vi "Main.vi"() -> ()   [LabVIEW 8.6]
uses:
  <vilib>/Analysis/NI_AALBase.lvlib
  <vilib>/Analysis/baseanly.llb/Mean (DBL).vi
panel:
  out "TemplateFilePath":path
  in  "Inspectors":string
  out "AvgValue":dbl
  out "CurveGraph":dbl[](graph)
  in  "Standard":string
  in  "SN":string
  in  "Type":string
  out "DateTime":timestamp format="%<%H:%M\n%Y/%m/%d>T"
  # "請看程式區說明"
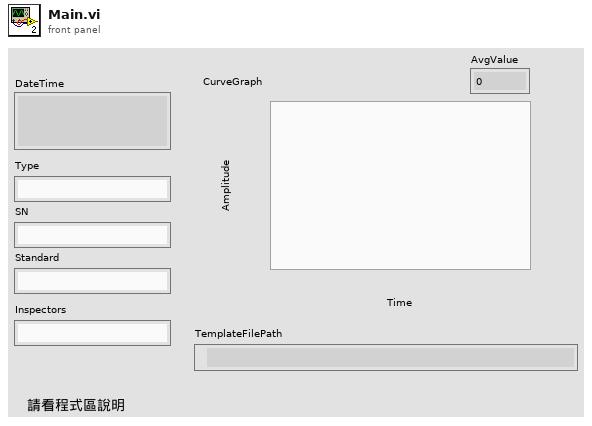
[diagram p1: front panel]
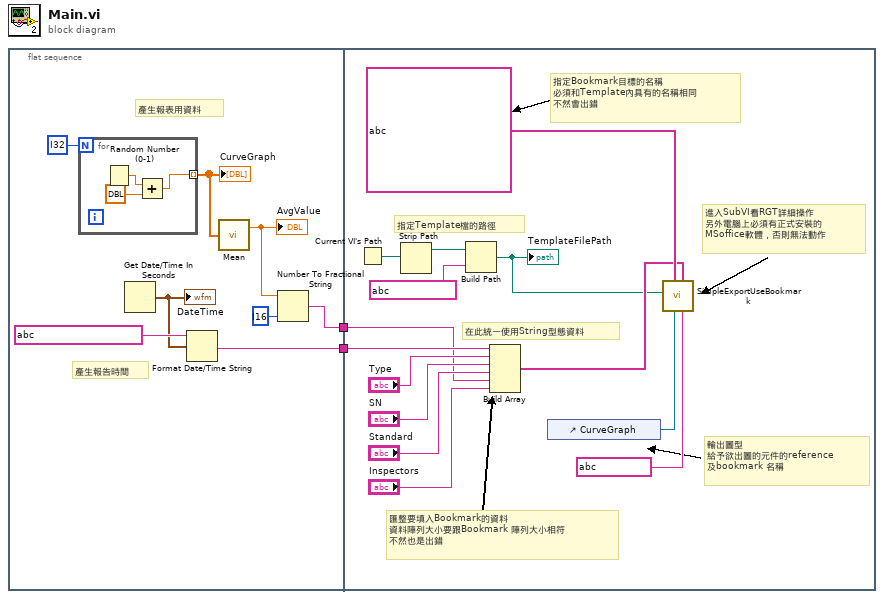
[diagram p0: block diagram]
diagram:
  n1 = flat-sequence {
    tunnel: [w4] -> w2
    tunnel: [w3] -> w1
    tunnel: w2 -> [w26]
    tunnel: w1 -> [w22]
    frame #0 {
      # "產生報告時間"
      # "產生報表用資料"
      n2 = for {
        N: i32 ? ("Numeric") -> [_]
        tunnel: [w11] -> w9 mode=indexing
        n3 = Random Number (0-1)() -> (number: 0 to 1=w13:dbl)
        n4 = Add(x=w13, y=dbl ?) -> (x+y=w11:dbl)
      }
      "CurveGraph" <- w9
      n5 = Get Date/Time In Seconds() -> (seconds since 1Jan1904=w7:timestamp)
      "DateTime" <- w7
      n6 = Format Date/Time String(time format string (%c)=string ?, seconds (now)=w7) -> (date/time string=w4:string)  [unwired: 1 in]
      n7 = call-poly <vilib>:"Mean.vi"("X"=w9) -> ("mean"=w6:dbl)  [unwired: 1 out]
      "AvgValue" <- w6
      n8 = Number To Fractional String(number=w6, precision (6)=i16 ?) -> (F-format string=w3:string)  [unwired: 2 in]
    }
    frame #1 {
      # "在此統一使用String型態資料"
      # "進入SubVI看RGT詳細操作\n另外電腦上必須有正式安裝的\nMSoffice軟體，否則無法動作"
      # "輸出圖型\n給予欲出圖的元件的reference\n及bookmark 名稱"
      # "匯整要填入Bookmark的資料\n資料陣列大小要跟Bookmark 陣列大小相符\n不然也是出錯"
      # "指定Bookmark目標的名稱\n必須和Template內具有的名稱相同\n不然會出錯"
      # "指定Template檔的路徑"
      n9 = Current VI's Path() -> (path=w17:path)
      n10 = Strip Path(path=w17) -> (stripped path=w16:path)  [unwired: 1 out]
      n11 = Build Path(base path=w16, name or relative path=string ?) -> (appended path=w14:path)
      "TemplateFilePath" <- w14
      n12 = Build Array(w26, "Type", "SN", "Standard", w22, "Inspectors") -> (w20:string[])
      n13 = control-ref of="CurveGraph"() -> (w19:refnum<vi>)
      n14 = call "SimpleExportUseBookmark.vi"("GraphBookmark"=string ?, "StringData"=w20, "GraphReference"=w19, "BookmarkTarget"=string[] ?, "TemplateFilePath"=w14) -> ()  [unwired: 6 in, 1 out]
    }
  }
